vi "ParseProcessErrorMessage.vi"(8 "error in (no error)":errorcluster, 11 "process error message":variant) -> (0 "error out":errorcluster, 2 "error string":string)   [LabVIEW 2017, in "Qbus.lvclass"]
uses:
  <vilib>/addons/Qbus/Qbus.lvclass
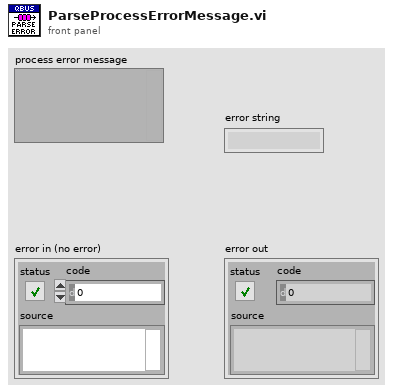
[diagram p1: front panel]
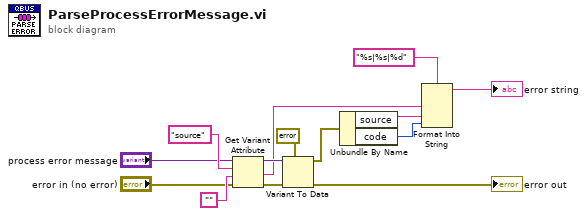
[diagram p0: block diagram]
diagram:
  n1 = Get Variant Attribute(Variant="process error message", name="source", default value (empty Variant)="", error in="error in (no error)") -> (duplicate Variant=w8:variant, value=w5:string, error out=w9:errorcluster)  [unwired: 1 out]
  n2 = Variant To Data(error in=w9, type=errorcluster {"status"=FALSE, "code"=0, "source"=""} ("error out"), Variant=w8) -> (data=w6:errorcluster, error out=→"error out":errorcluster)
  n3 = Unbundle By Name(w6) -> ("source"=w12:string, "code"=w11:i32)
  n4 = Format Into String(format string="%s|%s|%d", w5, w12, w11) -> (resulting string=→"error string":string)  [unwired: 2 in, 1 out]
